vi "DigUpPixAsync.vi"(7 "File Path":path, 9 "Result files to read":path[](array[path]), 11 "Cursor index":i32) -> ()   [LabVIEW 2022 SP3]
uses:
  b4501feb-eeb7-4aaa-9796-2bc830b7db41.vi
  0c3c7a91-34d3-4458-b7bc-66647a20b7f8.vi
  5db2d16c-fbaa-6048-903b-14ff5825f201.vi
  Anemometry/Anemometry Sub Vis/Globals/Constants_global.vi
panel:
  # "Remote Call to DigUpPix.vi, to make it non-blocking"
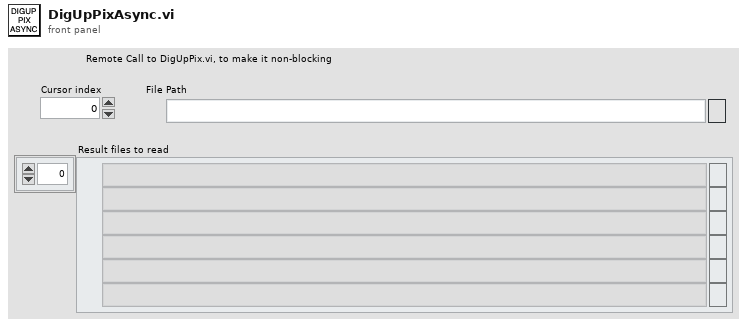
[diagram p1: front panel]
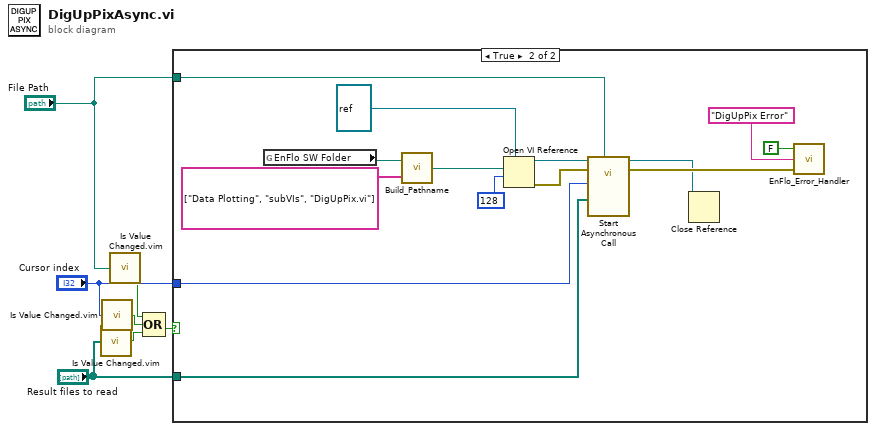
[diagram p0: block diagram]
diagram:
  n1 = call "Is Value Changed.vim"("value"="Result files to read") -> ("changed or first call?"=w3:bool)
  n2 = call "Is Value Changed.vim"("value"="Cursor index") -> ("changed or first call?"=w4:bool)
  n3 = call "Is Value Changed.vim"("value"="File Path") -> ("changed or first call?"=w1:bool)
  n4 = Compound Arithmetic op=OR(w1, w4, w3) -> (w2:bool)
  n5 = case shown="True" w2 {
    tunnel: "Cursor index" -> [_ w10]
    tunnel: "Result files to read" -> [_ w9]
    tunnel: "File Path" -> [_ w8]
    frame False {
    }
    frame True {
      n6 = global read "Constants_global.vi" "EnFlo SW Folder"() -> (w13:path)
      n7 = call "Build_Pathname.vi"("PathElements"=string[] ["Data Plotting", "subVIs", "DigUpPix.vi"] ("array of strings"), "PathnameIn"=w13) -> ("AppendedPath"=w21:path)
      n8 = Open VI Reference(type specifier VI Refnum (for type only)=refnum<vi> refnum, vi path=w21, options=128) -> (vi reference=w14:refnum<vi>, error out=w17:errorcluster)  [unwired: 3 in]
      n9 = call-by-ref "Start Asynchronous Call"(reference=w14, error in=w17, "File Path"=w8, "Result files to read"=w9, "Cursor index"=w10) -> (reference out=w11:refnum<vi>, error out=w18:errorcluster)  [unwired: 9 in]
      n10 = Close Reference(reference=w11) -> ()  [unwired: 1 in, 1 out]
      n11 = call "EnFlo_Error_Handler.vi"("error in (no error)"=w18, "Error Type"="DigUpPix Error", "Dialog Box (F)"=FALSE ("Dialog Box (T)")) -> ()  [unwired: 1 in, 2 out]
    }
  }
